vi "Loop_SM.vi"() -> ()   [LabVIEW 2017, in "Shooter.lvlib"]
uses:
  Shooter.lvlib
  Cluster_SM to HW Wheel Data.ctl
  Cluster_SM to HW Hood Data.ctl
  Cluster_CMD to SM Data.ctl
  ENUM_CMD Select.ctl
  TypeDefs/Cluster_SRX Status With Encoder.ctl
  TypeDefs/Cluster_SRX Limit Switches.ctl
  ENUM_State.ctl
  ENUM_Action.ctl
  Cluster_SM Status.ctl
  <vilib>/Rock Robotics/WPI/DriverStation/WPI_DriverStationRobotMode2.ctl
  Global_CMD to SM Data.vi
  Robot Global Data.vi
  Global_HW Status.vi
  Globals/Global_STOP.vi
  Sonar/Global_HW_Data Out.vi
  Controller/Global Control Outputs.vi
  Global_SM_Data Out.vi
  Sonar/Sonar.lvlib
  Controller/Controller.lvlib
panel:
  out "SM_Status OUT":T1
  in  "RPM Range":dbl=20.0
  out "Action":T2=enum."No Action"
  out "State":T3
  out "HW_Hood Limits":T4
  out "HW_Hood Status":T5
  out "HW_Wheel Status":T5
  out "CMD_Shooter":T6={"Select"=enum."Manual VBus", "Wheel VBus"=0.0, "Wheel RPM"=0.0, "Hood VBus"=0.0, "Hood Position"=0.0}
  out "Hood Data OUT":T8
  out "Wheel Data OUT":T9
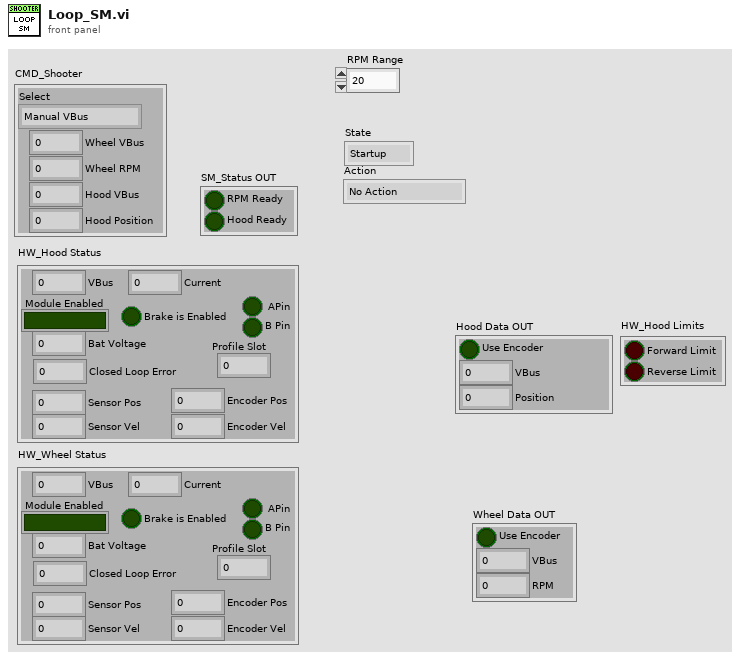
[diagram p1: front panel]
types:
  T1 = typedef "Shooter.lvlib/Cluster_SM Status.ctl" = cluster{"RPM Ready":bool, "Hood Ready":bool}
  T2 = typedef "Shooter.lvlib/ENUM_Action.ctl" = enum16{"Reset Compensations", "No Action", "Reset Time", "Reset All", "Set Wheel VBus", "Set Wheel RPM", "Set Hood VBus", "Set Hood Position", "Hood Stop"}
  T3 = typedef "Shooter.lvlib/ENUM_State.ctl" = enum16{"Startup", "Idle", "Shutdown", "Run", "Check Position", "Check Hopper", "Running"}
  T4 = typedef "Cluster_SRX Limit Switches.ctl" = cluster{"Forward Limit":bool, "Reverse Limit":bool}
  T5 = typedef "Cluster_SRX Status With Encoder.ctl" = cluster{"VBus ":dbl, "Module Enabled":bool, "Closed Loop Error":dbl, "Sensor Pos":dbl, "Sensor Vel":dbl, "Current":dbl, "Brake is Enabled":bool, "Encoder Pos":dbl, "Encoder Vel":dbl, " APin":bool, "B Pin":bool, "Bat Voltage":dbl, "Profile Slot":dbl}
  T6 = typedef "Shooter.lvlib/Cluster_CMD to SM Data.ctl" = cluster{"Select":T7, "Wheel VBus":dbl, "Wheel RPM":dbl, "Hood VBus":dbl, "Hood Position":dbl}
  T7 = typedef "Shooter.lvlib/ENUM_CMD Select.ctl" = enum16{"Stop", "Manual VBus", "Encoder Hood Only", "Encoder Wheel Only", "Encoder Both"}
  T8 = typedef "Shooter.lvlib/Cluster_SM to HW Hood Data.ctl" = cluster{"Use Encoder":bool, "VBus":dbl, "Position":dbl}
  T9 = typedef "Shooter.lvlib/Cluster_SM to HW Wheel Data.ctl" = cluster{"Use Encoder":bool, "VBus":dbl, "RPM":dbl}
  T10 = typedef "WPI_DriverStationRobotMode2.ctl" = enum16{"Autonomous Disabled", "Autonomous Enabled", "Teleop Disabled", "Teleop Enabled", "Disconnected", "Finish", "Test Disabled", "Test Enabled", "Emergency Stopped"}
  T11 = cluster{"Actions":T2[], "State":T3, "Current Time":timestamp, "Start Time":timestamp, "Loop Time (ms)":u32, "CMD Data":T6, "Robot Mode":T10, "Wheel Status ":T5, "Hood Status ":T5, "Wheel Data OUT":T9, "Hood Data OUT":T8, "Hood Limits":T4, "Sonar Distance":dbl, "Decrement Hood":bool, "Increment Hood":bool, "Increase RPM":bool, "Decrease RPM":bool, "Hood Compensation":dbl, "RPM Compensation":dbl, "SM_Status OUT":T1, "Start Time":timestamp}
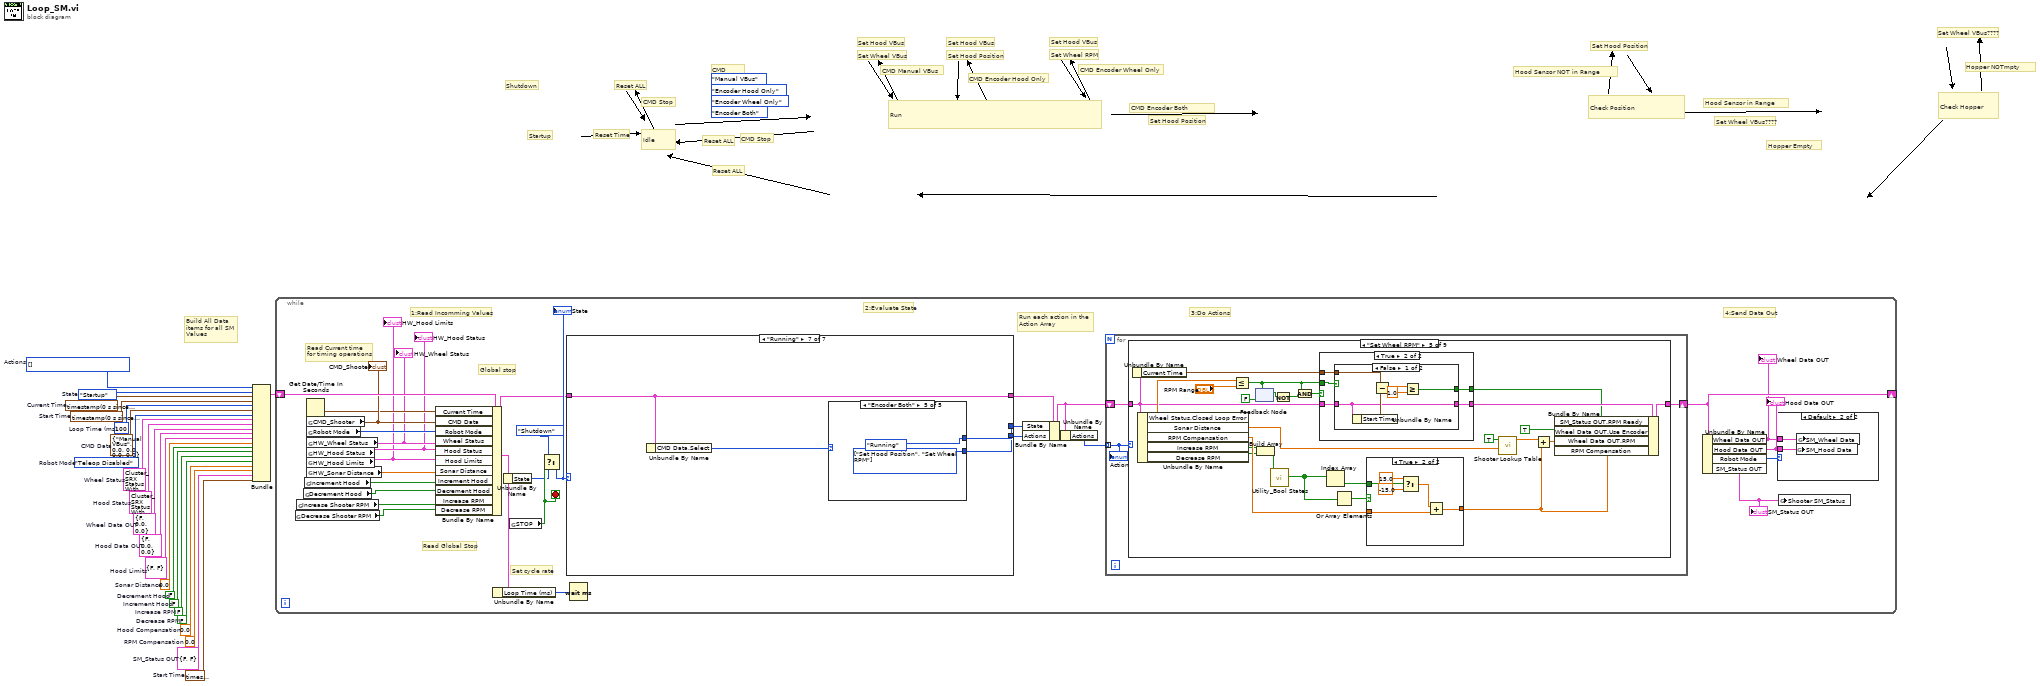
[diagram p0: block diagram]
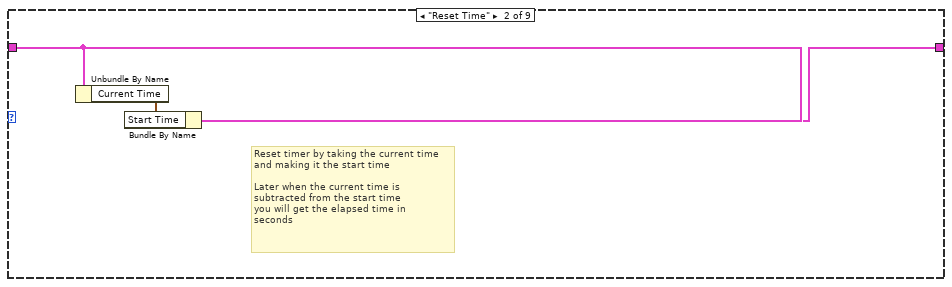
[diagram p4: hidden frame]
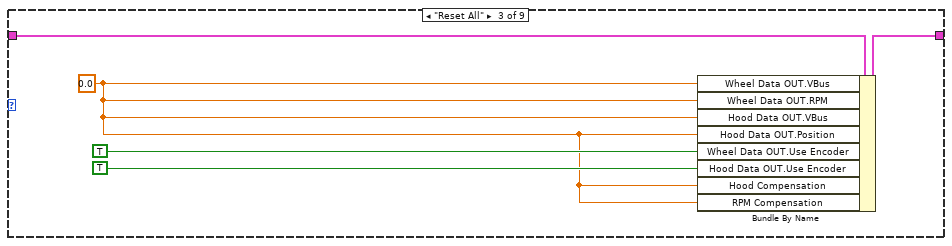
[diagram p5: hidden frame]
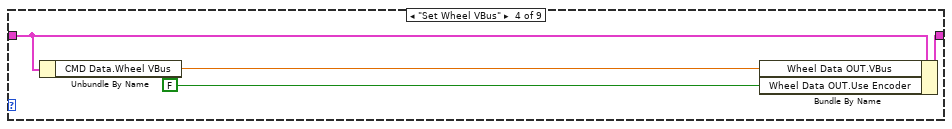
[diagram p6: hidden frame]
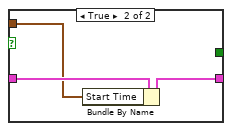
[diagram p8: hidden frame]
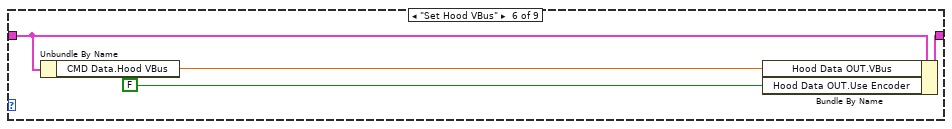
[diagram p10: hidden frame]
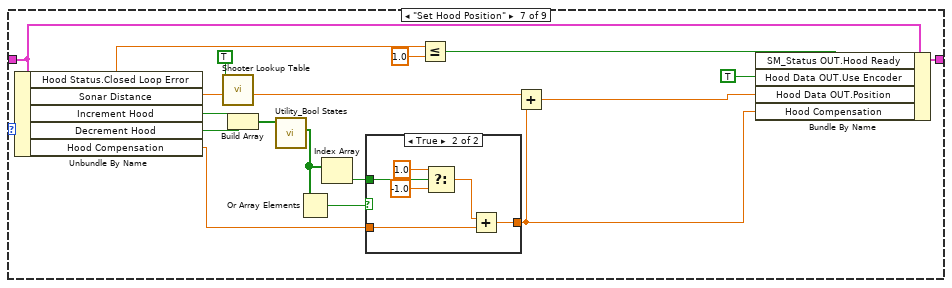
[diagram p11: hidden frame]
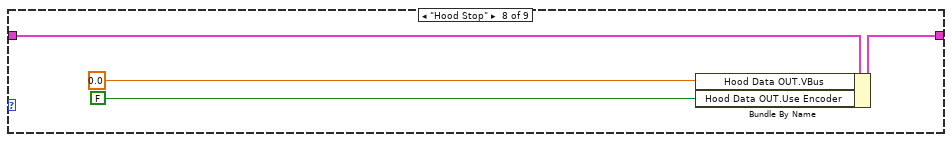
[diagram p13: hidden frame]
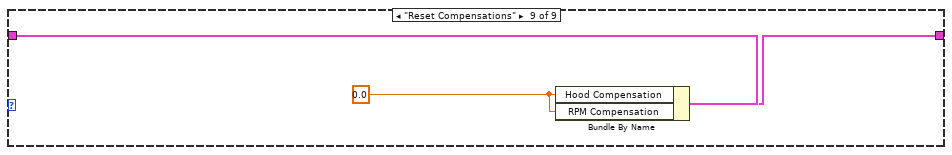
[diagram p14: hidden frame]
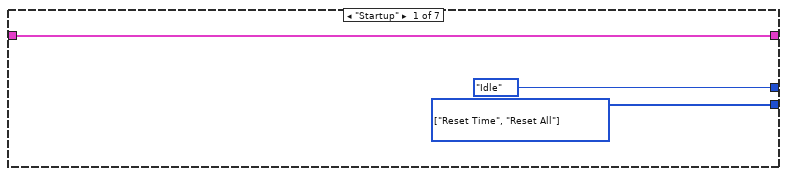
[diagram p15: hidden frame]
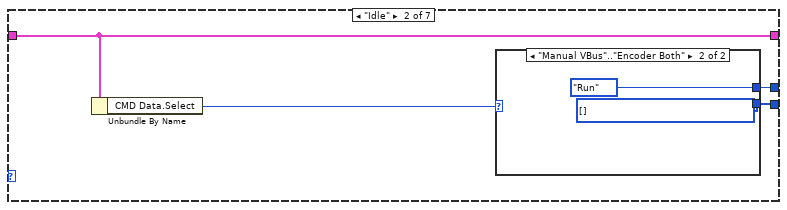
[diagram p16: hidden frame]
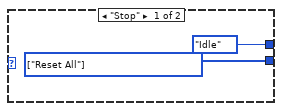
[diagram p17: hidden frame]
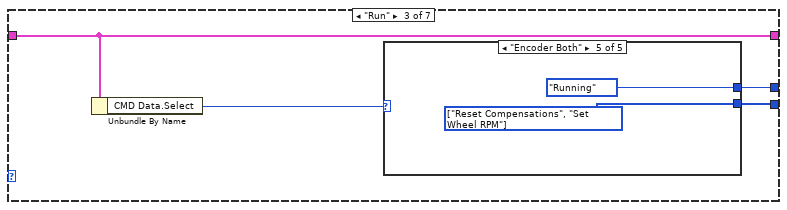
[diagram p18: hidden frame]
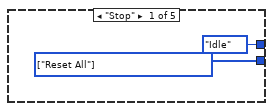
[diagram p19: hidden frame]
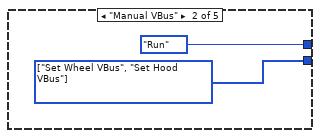
[diagram p20: hidden frame]
diagram:
  w1 = timestamp(0 s since 1904-01-01)  # Start Time
  w2 = T1 {"RPM Ready"=FALSE, "Hood Ready"=FALSE}  # SM_Status OUT
  w3 = 0.0  # RPM Compensation
  w4 = 0.0  # Hood Compensation
  w5 = FALSE  # Decrease RPM
  w6 = FALSE  # Increase RPM
  w7 = FALSE  # Increment Hood
  w8 = FALSE  # Decrement Hood
  w9 = 0.0  # Sonar Distance
  w10 = T4 {"Forward Limit"=FALSE, "Reverse Limit"=FALSE}  # Hood Limits
  w11 = T8 {"Use Encoder"=FALSE, "VBus"=0.0, "Position"=0.0}  # Hood Data OUT
  w12 = T9 {"Use Encoder"=FALSE, "VBus"=0.0, "RPM"=0.0}  # Wheel Data OUT
  w13 = T5 {"VBus "=0.0, "Module Enabled"=FALSE, "Closed Loop Error"=0.0, "Sensor Pos"=0.0, "Sensor Vel"=0.0, "Current"=0.0, "Brake is Enabled"=FALSE, "Encoder Pos"=0.0, "Encoder Vel"=0.0, " APin"=FALSE, "B Pin"=FALSE, "Bat Voltage"=0.0, "Profile Slot"=0.0}  # Hood Status
  w14 = T5 {"VBus "=0.0, "Module Enabled"=FALSE, "Closed Loop Error"=0.0, "Sensor Pos"=0.0, "Sensor Vel"=0.0, "Current"=0.0, "Brake is Enabled"=FALSE, "Encoder Pos"=0.0, "Encoder Vel"=0.0, " APin"=FALSE, "B Pin"=FALSE, "Bat Voltage"=0.0, "Profile Slot"=0.0}  # Wheel Status
  w15 = WPI_DriverStationRobotMode2."Teleop Disabled"  # Robot Mode
  (unwired) ENUM_CMD_Select."Encoder Both" ("CMD Data.Select")
  (unwired) ENUM_CMD_Select."Encoder Wheel Only" ("CMD Data.Select")
  (unwired) ENUM_CMD_Select."Encoder Hood Only" ("CMD Data.Select")
  (unwired) ENUM_CMD_Select."Manual VBus" ("CMD Data.Select")
  w16 = T6 {"Select"=enum."Manual VBus", "Wheel VBus"=0.0, "Wheel RPM"=0.0, "Hood VBus"=0.0, "Hood Position"=0.0}  # CMD Data
  w17 = u32 100  # Loop Time (ms)
  w18 = T2[] [] items=["Reset Compensations", "No Action", "Reset Time", "Reset All", "Set Wheel VBus", "Set Wheel RPM", "Set Hood VBus", "Set Hood Position", "Hood Stop"]  # Actions
  w19 = timestamp(0 s since 1904-01-01)  # Start Time
  w20 = timestamp(0 s since 1904-01-01)  # Current Time
  w21 = ENUM_State."Startup"  # State
  # "Set Wheel VBus????"
  # "Hopper NOTmpty"
  # "Hopper Empty"
  # "Reset ALL"
  # "Reset Time"
  # "Set Wheel VBus????"
  # "Set Hood Position"
  # "Hood Sensor NOT in Range"
  # "Hood Sensor in Range"
  # "Set Hood Position"
  # "CMD Encoder Both"
  # "Set Hood VBus"
  # "Set Wheel RPM"
  # "CMD Encoder Wheel Only"
  # "Set Hood VBus"
  # "Set Hood Position"
  # "CMD Encoder Hood Only"
  # "Set Hood VBus"
  # "Set Wheel VBus"
  # "CMD Manual VBus"
  # "Reset ALL"
  # "CMD Stop"
  # "CMD"
  # "Reset ALL"
  # "CMD Stop"
  # "Check Position"
  # "Run"
  # "Shutdown"
  # "Startup"
  # "Idle"
  # "Check Hopper"
  # "Build All Data items for all SM Values"
  n1 = Bundle("Actions"=w18, "State"=w21, "Current Time"=w20, "Start Time"=w19, "Loop Time (ms)"=w17, "CMD Data"=w16, "Robot Mode"=w15, "Wheel Status"=w14, "Hood Status"=w13, "Wheel Data OUT"=w12, "Hood Data OUT"=w11, "Hood Limits"=w10, "Sonar Distance"=w9, "Decrement Hood"=w8, "Increment Hood"=w7, "Increase RPM"=w6, "Decrease RPM"=w5, "Hood Compensation"=w4, "RPM Compensation"=w3, "SM_Status OUT"=w2, "Start Time"=w1) -> (w22:T11)  [unwired: 1 in]
  n2 = while {
    shift-right: [w40] -> _
    shift-left: w22 -> [w49]
    stop <- w44 stop-if-true
    # "Set cycle rate"
    # "Read Current time\nfor timing operations"
    # "Run each action in the Action Array"
    # "Read Global Stop"
    # "1:Read Incomming Values"
    # "2:Evaluate State"
    # "3:Do Actions"
    # "4:Send Data Out"
    # "Global stop"
    n3 = global read "Global Control Outputs.vi" "Decrease Shooter RPM"() -> (w24:bool)
    n4 = global read "Global Control Outputs.vi" "Increase Shooter RPM"() -> (w25:bool)
    n5 = global read "Global Control Outputs.vi" "Decrement Hood"() -> (w26:bool)
    n6 = global read "Global Control Outputs.vi" "Increment Hood"() -> (w27:bool)
    n7 = Get Date/Time In Seconds() -> (seconds since 1Jan1904=w36:timestamp)
    n8 = global read "Global_CMD to SM Data.vi" "CMD_Shooter"() -> (w37:T6)
    "CMD_Shooter" <- w37
    n9 = global read "Robot Global Data.vi" "Robot Mode"() -> (w35:T10)
    n10 = global read "Global_HW Status.vi" "HW_Wheel Status"() -> (w31:T5)
    "HW_Wheel Status" <- w31
    n11 = global read "Global_HW Status.vi" "HW_Hood Status"() -> (w30:T5)
    "HW_Hood Status" <- w30
    n12 = global read "Global_HW Status.vi" "HW_Hood Limits"() -> (w29:T4)
    "HW_Hood Limits" <- w29
    n13 = global read "Global_HW_Data Out.vi" "HW_Sonar Distance"() -> (w28:dbl)
    n14 = Bundle By Name(cluster=w49, "Current Time"=w36, "CMD Data"=w37, "Robot Mode"=w35, "Wheel Status"=w31, "Hood Status"=w30, "Hood Limits"=w29, "Sonar Distance"=w28, "Increment Hood"=w27, "Decrement Hood"=w26, "Increase RPM"=w25, "Decrease RPM"=w24) -> (w38:T11)
    n15 = Unbundle By Name(w38) -> ("Loop Time (ms)"=w39:u32)
    n16 = Unbundle By Name(w38) -> ("State"=w42:T3)
    n17 = global read "Global_STOP.vi" "STOP"() -> (w44:bool)
    n18 = Select(t=ENUM_State."Shutdown" ("State"), s=w44, f=w42) -> (s? t:f=w41:T3)
    "State" <- w41
    n19 = case shown="\"Running\"" w41 {
      tunnel: w38 -> [w154 w157 w165 w179 w187 w203 w205]
      tunnel: [w154 w157 w165 w179 w187 w203 w205] -> w47
      tunnel: [ENUM_State."Idle" ("State") w158 w166 ENUM_State."Shutdown" ("State") w189 ENUM_State."Check Hopper" ("State") w207] -> w46
      tunnel: [w153 w155 w163 w177 w188 w201 w206] -> w45
      frame "Startup" {
        w153 = T2[] [enum."Reset Time", enum."Reset All"] items=["Reset Compensations", "No Action", "Reset Time", "Reset All", "Set Wheel VBus", "Set Wheel RPM", "Set Hood VBus", "Set Hood Position", "Hood Stop"] ("Actions")
      }
      frame "Idle" {
        n20 = Unbundle By Name(w157) -> ("CMD Data.Select"=w156:T7)
        n21 = case shown="\"Manual VBus\"..\"Encoder Both\"" w156 {
          tunnel: [ENUM_State."Idle" ("State") ENUM_State."Run" ("State")] -> w158
          tunnel: [w159 w161] -> w155
          frame "Stop" {
            w159 = T2[] [enum."Reset All"] items=["Reset Compensations", "No Action", "Reset Time", "Reset All", "Set Wheel VBus", "Set Wheel RPM", "Set Hood VBus", "Set Hood Position", "Hood Stop"] ("Actions")
          }
          frame "Manual VBus".."Encoder Both" {
            w161 = T2[] [] items=["Reset Compensations", "No Action", "Reset Time", "Reset All", "Set Wheel VBus", "Set Wheel RPM", "Set Hood VBus", "Set Hood Position", "Hood Stop"] ("Actions")
          }
        }
      }
      frame "Run" {
        n22 = Unbundle By Name(w165) -> ("CMD Data.Select"=w164:T7)
        n23 = case shown="\"Encoder Both\"" w164 {
          tunnel: [ENUM_State."Idle" ("State") ENUM_State."Run" ("State") ENUM_State."Check Position" ("State") ENUM_State."Run" ("State") ENUM_State."Running" ("State")] -> w166
          tunnel: [w167 w169 w171 w173 w175] -> w163
          frame "Stop" {
            w167 = T2[] [enum."Reset All"] items=["Reset Compensations", "No Action", "Reset Time", "Reset All", "Set Wheel VBus", "Set Wheel RPM", "Set Hood VBus", "Set Hood Position", "Hood Stop"] ("Actions")
          }
          frame "Manual VBus" {
            w169 = T2[] [enum."Set Wheel VBus", enum."Set Hood VBus"] items=["Reset Compensations", "No Action", "Reset Time", "Reset All", "Set Wheel VBus", "Set Wheel RPM", "Set Hood VBus", "Set Hood Position", "Hood Stop"] ("Actions")
          }
          frame "Encoder Hood Only" {
            w171 = T2[] [enum."Set Hood Position", enum."Set Wheel VBus"] items=["Reset Compensations", "No Action", "Reset Time", "Reset All", "Set Wheel VBus", "Set Wheel RPM", "Set Hood VBus", "Set Hood Position", "Hood Stop"] ("Actions")
          }
          frame "Encoder Wheel Only" {
            w173 = T2[] [enum."Set Wheel RPM", enum."Set Hood VBus"] items=["Reset Compensations", "No Action", "Reset Time", "Reset All", "Set Wheel VBus", "Set Wheel RPM", "Set Hood VBus", "Set Hood Position", "Hood Stop"] ("Actions")
          }
          frame "Encoder Both" {
            w175 = T2[] [enum."Reset Compensations", enum."Set Wheel RPM"] items=["Reset Compensations", "No Action", "Reset Time", "Reset All", "Set Wheel VBus", "Set Wheel RPM", "Set Hood VBus", "Set Hood Position", "Hood Stop"] ("Actions")
          }
        }
      }
      frame "Shutdown" {
        w177 = T2[] [enum."Reset All"] items=["Reset Compensations", "No Action", "Reset Time", "Reset All", "Set Wheel VBus", "Set Wheel RPM", "Set Hood VBus", "Set Hood Position", "Hood Stop"] ("Actions")
      }
      frame "Check Position" {
        n24 = Unbundle By Name(w187) -> ("CMD Data.Hood Position"=w186:dbl, "Hood Status.Sensor Pos"=w185:dbl, "CMD Data.Select"=w180:T7)
        n25 = Subtract(x=w186, y=w185) -> (x-y=w184:dbl)
        n26 = In Range and Coerce(upper limit=0.05, x=w184, lower limit=-0.05) -> (In Range?=w181:bool)  [unwired: 1 out]
        n27 = case shown="True" w181 {
          tunnel: [ENUM_State."Check Position" ("State") w193] -> w189
          tunnel: [w190 w192] -> w188
          tunnel: w180 -> [_ w194]
          frame False {
            w190 = T2[] [enum."Set Hood Position", enum."Set Wheel VBus"] items=["Reset Compensations", "No Action", "Reset Time", "Reset All", "Set Wheel VBus", "Set Wheel RPM", "Set Hood VBus", "Set Hood Position", "Hood Stop"] ("Actions")
          }
          frame True {
            n28 = case shown="\"Encoder Both\"" w194 {
              tunnel: [ENUM_State."Running" ("State") ENUM_State."Idle" ("State") ENUM_State."Running" ("State")] -> w193
              tunnel: [w195 w197 w199] -> w192
              frame "Encoder Hood Only", Default {
                w195 = T2[] [enum."Hood Stop", enum."Set Wheel VBus"] items=["Reset Compensations", "No Action", "Reset Time", "Reset All", "Set Wheel VBus", "Set Wheel RPM", "Set Hood VBus", "Set Hood Position", "Hood Stop"] ("Actions")
              }
              frame "Stop" {
                w197 = T2[] [enum."Reset All"] items=["Reset Compensations", "No Action", "Reset Time", "Reset All", "Set Wheel VBus", "Set Wheel RPM", "Set Hood VBus", "Set Hood Position", "Hood Stop"] ("Actions")
              }
              frame "Encoder Both" {
                w199 = T2[] [enum."Hood Stop", enum."Set Wheel RPM"] items=["Reset Compensations", "No Action", "Reset Time", "Reset All", "Set Wheel VBus", "Set Wheel RPM", "Set Hood VBus", "Set Hood Position", "Hood Stop"] ("Actions")
              }
            }
          }
        }
      }
      frame "Check Hopper" {
        w201 = T2[] [enum."Set Wheel VBus", enum."Hood Stop"] items=["Reset Compensations", "No Action", "Reset Time", "Reset All", "Set Wheel VBus", "Set Wheel RPM", "Set Hood VBus", "Set Hood Position", "Hood Stop"] ("Actions")
      }
      frame "Running" {
        n29 = Unbundle By Name(w205) -> ("CMD Data.Select"=w204:T7)
        n30 = case shown="\"Encoder Both\"" w204 {
          tunnel: [ENUM_State."Idle" ("State") ENUM_State."Shutdown" ("State") ENUM_State."Running" ("State") ENUM_State."Startup" ("State") ENUM_State."Running" ("State")] -> w207
          tunnel: [w208 w210 w212 w214 w216] -> w206
          frame "Stop" {
            w208 = T2[] [enum."Reset All"] items=["Reset Compensations", "No Action", "Reset Time", "Reset All", "Set Wheel VBus", "Set Wheel RPM", "Set Hood VBus", "Set Hood Position", "Hood Stop"] ("Actions")
          }
          frame "Manual VBus" {
            w210 = T2[] [enum."Reset All"] items=["Reset Compensations", "No Action", "Reset Time", "Reset All", "Set Wheel VBus", "Set Wheel RPM", "Set Hood VBus", "Set Hood Position", "Hood Stop"] ("Actions")
          }
          frame "Encoder Hood Only" {
            w212 = T2[] [enum."Hood Stop", enum."Set Wheel VBus"] items=["Reset Compensations", "No Action", "Reset Time", "Reset All", "Set Wheel VBus", "Set Wheel RPM", "Set Hood VBus", "Set Hood Position", "Hood Stop"] ("Actions")
          }
          frame "Encoder Wheel Only" {
            w214 = T2[] [] items=["Reset Compensations", "No Action", "Reset Time", "Reset All", "Set Wheel VBus", "Set Wheel RPM", "Set Hood VBus", "Set Hood Position", "Hood Stop"] ("Actions")
          }
          frame "Encoder Both" {
            w216 = T2[] [enum."Set Hood Position", enum."Set Wheel RPM"] items=["Reset Compensations", "No Action", "Reset Time", "Reset All", "Set Wheel VBus", "Set Wheel RPM", "Set Hood VBus", "Set Hood Position", "Hood Stop"] ("Actions")
          }
        }
      }
    }
    n31 = Wait (ms)(milliseconds to wait=w39) -> ()  [unwired: 1 out]
    n32 = Bundle By Name(cluster=w47, "State"=w46, "Actions"=w45) -> (w48:T11)
    n33 = Unbundle By Name(w48) -> ("Actions"=w50:T2[])
    n34 = for {
      tunnel: w50 -> [w55] mode=indexing
      shift-right: [w54] -> w40
      shift-left: w48 -> [w53]
      n35 = case shown="\"Set Wheel RPM\"" w55 {
        tunnel: w53 -> [w56 w59 w64 w67 w74 w118 w136 w148 w151]
        tunnel: [w56 w58 w63 w68 w93 w119 w137 w147 w150] -> w54
        frame "No Action" {
        }
        frame "Reset Time" {
          # "Reset timer by taking the current time\nand making it the start time\n\nLater when the current time is \nsubtracted from the start time\nyou will get the elapsed time in \nseconds"
          n36 = Unbundle By Name(w59) -> ("Current Time"=w57:timestamp)
          n37 = Bundle By Name(cluster=w59, "Start Time"=w57) -> (w58:T11)
        }
        frame "Reset All" {
          w60 = 0.0 ("FG Write Value")
          n38 = Bundle By Name(cluster=w64, "Wheel Data OUT.VBus"=w60, "Wheel Data OUT.RPM"=w60, "Hood Data OUT.VBus"=w60, "Hood Data OUT.Position"=w60, "Wheel Data OUT.Use Encoder"=TRUE ("Wheel Encoder Out"), "Hood Data OUT.Use Encoder"=TRUE ("Hood Encoder Out"), "Hood Compensation"=w60, "RPM Compensation"=w60) -> (w63:T11)
        }
        frame "Set Wheel VBus" {
          n39 = Unbundle By Name(w67) -> ("CMD Data.Wheel VBus"=w66:dbl)
          n40 = Bundle By Name(cluster=w67, "Wheel Data OUT.VBus"=w66, "Wheel Data OUT.Use Encoder"=FALSE ("Wheel Encoder Out")) -> (w68:T11)
        }
        frame "Set Wheel RPM" {
          n41 = Unbundle By Name(w74) -> ("Current Time"=w71:timestamp)
          n42 = Unbundle By Name(w74) -> ("Wheel Status.Closed Loop Error"=w79:dbl, "Sonar Distance"=w91:dbl, "RPM Compensation"=w85:dbl, "Increase RPM"=w83:bool, "Decrease RPM"=w82:bool)
          n43 = Less Or Equal?(x=w79, y="RPM Range") -> (x <= y?=w72:bool)
          n44 = feedback-in #1(w72) -> ()
          n45 = feedback #1(FALSE) -> (w77:bool)
          n46 = Build Array(w83, w82) -> (w84:bool[])
          n47 = call "Utility_Bool States.vi"("HW_Joystick_Buttons"=w84) -> ("Rizing Out"=w81:bool[])  [unwired: 6 in, 4 out]
          n48 = Not(x=w77) -> (.not. x?=w76:bool)
          n49 = And(x=w72, y=w76) -> (x .and. y?=w75:bool)
          n50 = case shown="True" w75 {
            tunnel: w74 -> [w94 w98]
            tunnel: [w94 w97] -> w73
            tunnel: w72 -> [_ w99]
            tunnel: w71 -> [_ w96]
            tunnel: [_ w95] -> w70
            frame False {
            }
            frame True {
              n51 = case shown="False" w99 {
                tunnel: w98 -> [w101 w108]
                tunnel: [w101 w107] -> w97
                tunnel: w96 -> [w105 w106]
                tunnel: [w100 _] -> w95
                frame False {
                  n52 = Unbundle By Name(w101) -> ("Start Time"=w104:timestamp)
                  n53 = Subtract(x=w105, y=w104) -> (x-y=w103:dbl)
                  n54 = Greater Or Equal?(x=w103, y=1.0) -> (x >= y?=w100:bool)
                }
                frame True {
                  n55 = Bundle By Name(cluster=w108, "Start Time"=w106) -> (w107:T11)
                }
              }
            }
          }
          n56 = Index Array(array=w81) -> (element=w88:bool)  [unwired: 1 in]
          n57 = Or Array Elements(Boolean array=w81) -> (logical OR=w89:bool)
          n58 = case shown="True" w89 {
            tunnel: w85 -> [w109 w113]
            tunnel: [w109 w111] -> w87
            tunnel: w88 -> [_ w110]
            frame False {
            }
            frame True {
              n59 = Select(t=15.0, s=w110, f=-15.0) -> (s? t:f=w112:dbl)
              n60 = Add(x=w112, y=w113) -> (x+y=w111:dbl)
            }
          }
          n61 = call "Shooter Lookup Table.vi"("Sonar Value"=w91, "Final(t) Slop(f)"=TRUE ("Final(t) Slot(f)")) -> ("RPM"=w86:dbl)  [unwired: 8 in, 1 out]
          n62 = Add(x=w86, y=w87) -> (x+y=w80:dbl)
          n63 = Bundle By Name(cluster=w73, "SM_Status OUT.RPM Ready"=w70, "Wheel Data OUT.Use Encoder"=TRUE ("Wheel Encoder Out"), "Wheel Data OUT.RPM"=w80, "RPM Compensation"=w87) -> (w93:T11)
        }
        frame "Set Hood VBus" {
          n64 = Unbundle By Name(w118) -> ("CMD Data.Hood VBus"=w117:dbl)
          n65 = Bundle By Name(cluster=w118, "Hood Data OUT.VBus"=w117, "Hood Data OUT.Use Encoder"=FALSE ("Wheel Encoder Out")) -> (w119:T11)
        }
        frame "Set Hood Position" {
          n66 = Unbundle By Name(w136) -> ("Hood Status.Closed Loop Error"=w122:dbl, "Sonar Distance"=w133:dbl, "Increment Hood"=w128:bool, "Decrement Hood"=w127:bool, "Hood Compensation"=w132:dbl)
          n67 = call "Shooter Lookup Table.vi"("Sonar Value"=w133, "Final(t) Slop(f)"=TRUE ("Final(t) Slot(f)")) -> ("Hood"=w131:dbl)  [unwired: 8 in, 1 out]
          n68 = Build Array(w128, w127) -> (w126:bool[])
          n69 = call "Utility_Bool States.vi"("HW_Joystick_Buttons"=w126) -> ("Rizing Out"=w123:bool[])  [unwired: 6 in, 4 out]
          n70 = Or Array Elements(Boolean array=w123) -> (logical OR=w125:bool)
          n71 = Index Array(array=w123) -> (element=w124:bool)  [unwired: 1 in]
          n72 = case shown="True" w125 {
            tunnel: w132 -> [w138 w142]
            tunnel: [w138 w140] -> w129
            tunnel: w124 -> [_ w139]
            frame False {
            }
            frame True {
              n73 = Select(t=1.0, s=w139, f=-1.0) -> (s? t:f=w141:dbl)
              n74 = Add(x=w141, y=w142) -> (x+y=w140:dbl)
            }
          }
          n75 = Less Or Equal?(x=w122, y=1.0) -> (x <= y?=w120:bool)
          n76 = Add(x=w131, y=w129) -> (x+y=w130:dbl)
          n77 = Bundle By Name(cluster=w136, "SM_Status OUT.Hood Ready"=w120, "Hood Data OUT.Use Encoder"=TRUE ("Wheel Encoder Out"), "Hood Data OUT.Position"=w130, "Hood Compensation"=w129) -> (w137:T11)
        }
        frame "Hood Stop" {
          n78 = Bundle By Name(cluster=w148, "Hood Data OUT.VBus"=0.0 ("Hood VBus Out"), "Hood Data OUT.Use Encoder"=FALSE ("Hood Encoder Out")) -> (w147:T11)
        }
        frame "Reset Compensations" {
          w149 = 0.0 ("Hood Compensation")
          n79 = Bundle By Name(cluster=w151, "Hood Compensation"=w149, "RPM Compensation"=w149) -> (w150:T11)
        }
      }
      "Action" <- w55
    }
    n80 = Unbundle By Name(w40) -> ("Wheel Data OUT"=w32:T9, "Hood Data OUT"=w33:T8, "Robot Mode"=w34:T10, "SM_Status OUT"=w23:T1)
    "Wheel Data OUT" <- w32
    "Hood Data OUT" <- w33
    "SM_Status OUT" <- w23
    n81 = case shown="Default" w34 {
      tunnel: w33 -> [_ w51]
      tunnel: w32 -> [_ w52]
      frame "Test Enabled" {
      }
      frame Default {
        n82 = global write "Global_SM_Data Out.vi" "SM_Hood Data"(w51) -> ()
        n83 = global write "Global_SM_Data Out.vi" "SM_Wheel Data"(w52) -> ()
      }
    }
    n84 = global write "Global_SM_Data Out.vi" "Shooter SM_Status"(w23) -> ()
  }
